vi "Options_Statistics.vi"() -> (3 "Array_Int_OUT":i32[](array[numeric]))   [LabVIEW 2020]
doc: "Za pomocą polecenia SQL umieszcza w tablicy krotoność wybieranych opcji."
uses:
  <vilib>/drjdpowell/SQLite Library/SQL Connection/Open (path).vi
  <vilib>/drjdpowell/SQLite Library/SQL Connection/Open (string).vi
  <vilib>/AdvancedString/Path To Command Line String.vi
  <vilib>/drjdpowell/SQLite Library/SQL Connection/Execute SQL (Single String).vi
  <vilib>/drjdpowell/SQLite Library/SQL Connection/Connection.lvclass
  <vilib>/drjdpowell/SQLite Library/SQLite.lvlib
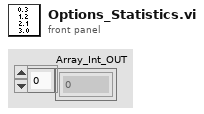
[diagram p1: front panel]
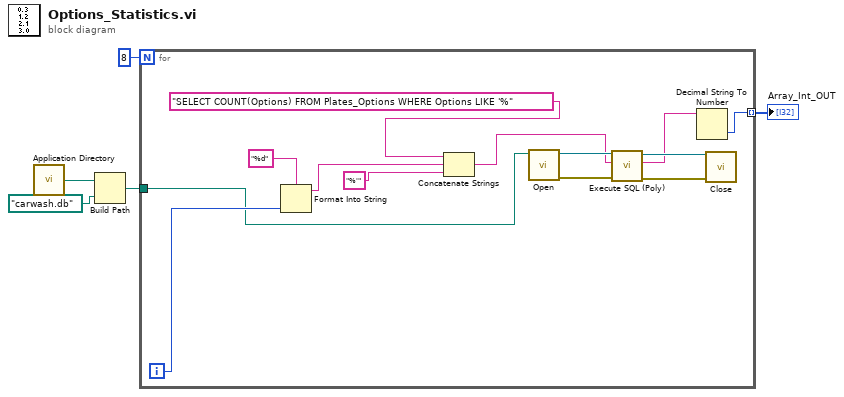
[diagram p0: block diagram]
diagram:
  n1 = call <vilib>:"Application Directory.vi"() -> ("Application Directory"=w4:path)
  n2 = Build Path(base path=w4, name or relative path=path "carwash.db" ("db file")) -> (appended path=w2:path)
  n3 = for {
    N: 8 -> [_]
    tunnel: [w6] -> w1 mode=indexing
    tunnel: w2 -> [w8]
    i -> [w10]
    n4 = Format Into String(format string="%d", w10) -> (resulting string=w14:string)  [unwired: 2 in, 1 out]
    n5 = Concatenate Strings("SELECT COUNT(Options) FROM Plates_Options WHERE Options LIKE '%", w14, "%'" ("SQL")) -> (w11:string)
    n6 = call-poly <vilib>:"Open.vi"("db file"=w8) -> ("error out"=w17:errorcluster, "SQLite Connection"=w18:refnum<class "Connection.lvclass">)  [unwired: 9 in]
    n7 = call-poly <vilib>:"Execute SQL (Poly).vi"("error in (no error)"=w17, "SQL"=w11, "SQLite Connection in"=w18) -> ("error out"=w16:errorcluster, "Result"=w7:string, "SQLite Connection"=w15:refnum<class "Connection.lvclass">)  [unwired: 6 in]
    n8 = Decimal String To Number(string=w7) -> (number=w6:i32)  [unwired: 2 in, 1 out]
    n9 = call-dynamic "Close.vi"("error in (no error)"=w16, "SQLite Connection in"=w15) -> ()  [unwired: 9 in, 1 out]
  }
  "Array_Int_OUT" <- w1
